vi "Scale Color TB.vi"() -> ()   [LabVIEW 2013]
panel:
  out "Color Out":u32(colorbox)
  out "Output Bght":u8
  out "Input Bght":u8
  in  "Color In":u32(colorbox)
  in  "Brightness":u8
  in  "Factor":dbl
  in  "stop":bool
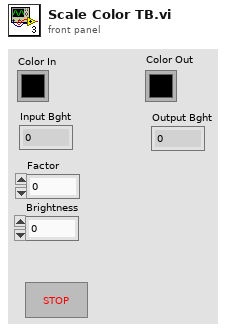
[diagram p1: front panel]
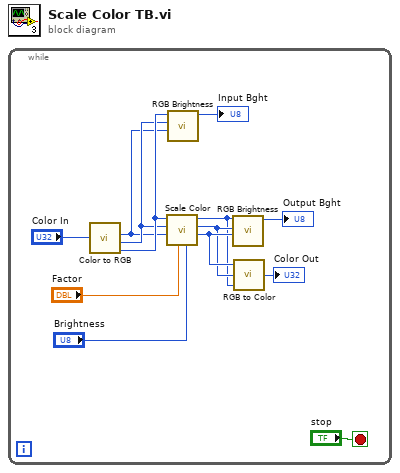
[diagram p0: block diagram]
diagram:
  n1 = while {
    stop <- "stop" stop-if-true
    n2 = call <vilib>:"Color to RGB.vi"("Color"="Color In") -> ("R"=w7:u8, "G"=w8:u8, "B"=w9:u8)  [unwired: 1 out]
    n3 = call "Scale Color.vi"("Brightness"="Brightness", "Factor"="Factor", "Red"=w7, "Green"=w8, "Blue"=w9) -> ("Red Out"=w4:u8, "Green Out"=w3:u8, "Blue Out"=w2:u8)  [unwired: 4 in]
    n4 = call "RGB Brightness.vi"("Red"=w7, "Green"=w8, "Blue"=w9) -> ("Brightness"=→"Input Bght":u8)  [unwired: 8 in]
    n5 = call "RGB Brightness.vi"("Red"=w4, "Green"=w3, "Blue"=w2) -> ("Brightness"=→"Output Bght":u8)  [unwired: 8 in]
    n6 = call <vilib>:"RGB to Color.vi"("B"=w2, "G"=w3, "R"=w4) -> ("Color"=→"Color Out":u32)
  }
